vi "Instr_InitObject.vi"(8 "error in (no error)":errorcluster, 9 "Instrument Configuration":variant, 10 "GPIB address":string, 11 "KE2410 in":refnum<class "KE2410.lvclass">) -> (0 "error out":errorcluster, 3 "KE2410 out":refnum<class "KE2410.lvclass">)   [LabVIEW 2018, in "KE2410.lvclass"]
uses:
  KE2410.lvclass
  InstrumentSetup.vi
  KE2410_CommandsGlobal.vi
  SupplyControl.lvclass
  InstrControl.lvclass
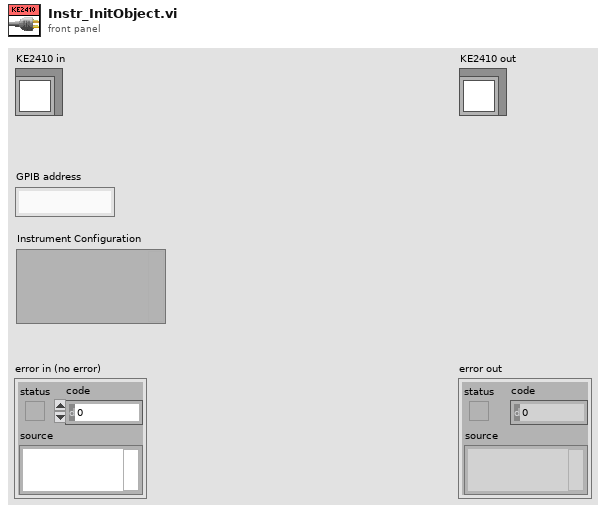
[diagram p1: front panel]
types:
  T1 = cluster{"Current Limit":sgl, "KE2410":refnum<class "KE2410.lvclass">}
  T2 = cluster{"Instrument name":string, "Command \"Reset\"":string, "Command \"Initialise\"":string, "Command \"Arm\"":string, "Command \"SetVolts\"":string, "Command \"Compliance?\"":string, "Command \"Standby\"":string, "Command \"Read Current\"":string}
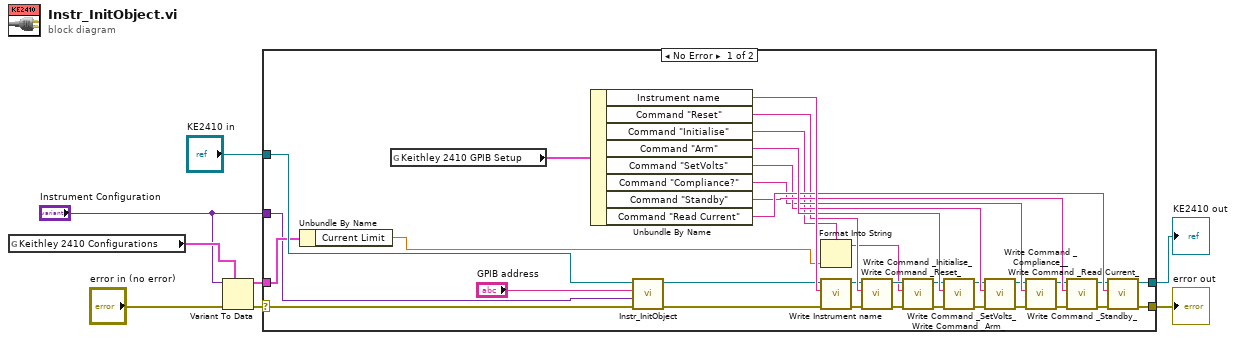
[diagram p0: block diagram]
diagram:
  n1 = global read "InstrumentSetup.vi" "Keithley 2410 Configurations"() -> (w4:T1)
  n2 = Variant To Data(error in="error in (no error)", type=w4, Variant="Instrument Configuration") -> (data=w5:T1, error out=w2:errorcluster)
  n3 = case shown="No Error" w2 {
    selector: w2 -> [w14 w44]
    tunnel: [w22 w44] -> w8
    tunnel: [w23 w43] -> w6
    tunnel: "KE2410 in" -> [w16 w43]
    tunnel: w5 -> [w11 _]
    tunnel: "Instrument Configuration" -> [w10 _]
    frame No Error {
      n4 = Unbundle By Name(w11) -> ("Current Limit"=w21:sgl)
      n5 = global read "KE2410_CommandsGlobal.vi" "Keithley 2410 GPIB Setup"() -> (w9:T2)
      n6 = Unbundle By Name(w9) -> ("Instrument name"=w42:string, "Command \"Reset\""=w36:string, "Command \"Initialise\""=w20:string, "Command \"Arm\""=w41:string, "Command \"SetVolts\""=w38:string, "Command \"Compliance?\""=w37:string, "Command \"Standby\""=w39:string, "Command \"Read Current\""=w40:string)
      n7 = call-parent "Instr_InitObject.vi"("error in (no error)"=w14, "Instrument Configuration"=w10, "GPIB address"="GPIB address", "SupplyControl in"=w16) -> ("error out"=w13:errorcluster, "SupplyControl out"=w15:refnum<class "KE2410.lvclass">)  [unwired: 6 in]
      n8 = Format Into String(format string=w20, w21) -> (resulting string=w19:string)  [unwired: 2 in, 1 out]
      n9 = call-dynamic "Write Instrument name.vi"("error in (no error)"=w13, "Instrument name"=w42, "InstControl in"=w15) -> ("error out"=w17:errorcluster, "InstControl out"=w18:refnum<class "KE2410.lvclass">)  [unwired: 7 in]
      n10 = call-dynamic "Write Command _Reset_.vi"("error in (no error)"=w17, "Command \"Reset\""=w36, "SupplyControl in"=w18) -> ("error out"=w29:errorcluster, "SupplyControl out"=w35:refnum<class "KE2410.lvclass">)  [unwired: 7 in]
      n11 = call-dynamic "Write Command _Initialise_.vi"("error in (no error)"=w29, "Command \"Initialise\""=w19, "SupplyControl in"=w35) -> ("error out"=w28:errorcluster, "SupplyControl out"=w34:refnum<class "KE2410.lvclass">)  [unwired: 7 in]
      n12 = call-dynamic "Write Command _Arm_.vi"("error in (no error)"=w28, "Command \"Arm\""=w41, "SupplyControl in"=w34) -> ("error out"=w27:errorcluster, "SupplyControl out"=w33:refnum<class "KE2410.lvclass">)  [unwired: 7 in]
      n13 = call-dynamic "Write Command _SetVolts_.vi"("error in (no error)"=w27, "Command \"SetVolts\""=w38, "SupplyControl in"=w33) -> ("error out"=w26:errorcluster, "SupplyControl out"=w32:refnum<class "KE2410.lvclass">)  [unwired: 7 in]
      n14 = call-dynamic "Write Command _Compliance__.vi"("error in (no error)"=w26, "Command \"Compliance?\""=w37, "SupplyControl in"=w32) -> ("error out"=w25:errorcluster, "SupplyControl out"=w31:refnum<class "KE2410.lvclass">)  [unwired: 7 in]
      n15 = call-dynamic "Write Command _Standby_.vi"("error in (no error)"=w25, "Command \"Standby\""=w39, "SupplyControl in"=w31) -> ("error out"=w24:errorcluster, "SupplyControl out"=w30:refnum<class "KE2410.lvclass">)  [unwired: 7 in]
      n16 = call-dynamic "Write Command _Read Current_.vi"("error in (no error)"=w24, "Command \"Read Current\""=w40, "SupplyControl in"=w30) -> ("error out"=w22:errorcluster, "SupplyControl out"=w23:refnum<class "KE2410.lvclass">)  [unwired: 7 in]
    }
    frame Error {
    }
  }
  "error out" <- w8
  "KE2410 out" <- w6
